vi "Grid_Move_to_point.vi"(6 "point":i64, 9 "FileRefs in":T1, 10 "Settings":T2={"Drift Correction Settings"={"Drift Correction every"=80, "Drift correction Pixels"=256, "Channel index (0-23)"=0, "MaxImagesBack"=2, "Threshold"=2, "Increment"=8, "max applied Drift Correction"=20, "Correct Drift"=TRUE, "Correlate"=0, "Correct z drift"=FALSE, "zdrift \nDuration (s)"=0.0}, "Spectroscopy Setting"={"Imaging Current"=1e-11, "ref Current"=7e-11, "tip Speed (m/s)"=2e-09, "Imaging Bias"=0.02, "ref Bias"=-0.1, "preSTS delay [ms]"=500, "STS z offset"=2e-10, "during Spec Bias (V)"=-0.1, "trigger1 < Hz"=0.0, "trigger 2 >Hz"=0.0, "autoStop"=FALSE, "Spectroscopy"=0, "PLL ON/OFF"=TRUE, "readjust setpoint every "=1, "z Reference"=FALSE, "Lock In"=TRUE}, "Misc"={"File name"="symmetric_node_zOff=200p", "Email when finished"="cornelius.krull@monash.edu,Dhaneesh.Gopalakrishnan@monash.edu,marina.castelli@monash.edu"}, "Grid Settings"={"type"=1, "type order"=1, "X pixel"=0, "Y pixel"=0, "Grid_Parms"={"center X (m)"=0.0, "center Y (m)"=0.0, "width (m)"=0.0, "height (m)"=0.0, "angle (deg)"=0.0}}} {"Grid Settings"."type order" items=["Line", "Grid"]; "Grid Settings"."type" items=["Line", "Grid"]; "Spectroscopy Setting"."Spectroscopy" items=["Bias", "zSpec"]; "Spectroscopy Setting"."trigger 2 >Hz" format="%#_6p"; "Spectroscopy Setting"."trigger1 < Hz" format="%#_6p"; "Spectroscopy Setting"."during Spec Bias (V)" format="%#_5p"; "Spectroscopy Setting"."STS z offset" format="%#_6p"; "Spectroscopy Setting"."ref Bias" format="%#_6p"; "Spectroscopy Setting"."Imaging Bias" format="%#_6p"; "Spectroscopy Setting"."tip Speed (m/s)" format="%.2p"; "Spectroscopy Setting"."ref Current" format="%#_6p"; "Spectroscopy Setting"."Imaging Current" format="%#_6p"; "Drift Correction Settings"."Correlate" items=["first Frame", "successive Frames"]; "Drift Correction Settings"."max applied Drift Correction" min=1 max=100 step=1 format="%.0p"; "Drift Correction Settings"."Threshold" min=1 step=1; "Drift Correction Settings"."Channel index (0-23)" items=["Current"=0, "Z (m)"=14]}, 11 "Application ref in":refnum<vi>) -> (1 "FileRefs out":T1, 2 "Settings out":T2={"Drift Correction Settings"={"Drift Correction every"=80, "Drift correction Pixels"=256, "Channel index (0-23)"=0, "MaxImagesBack"=2, "Threshold"=2, "Increment"=8, "max applied Drift Correction"=20, "Correct Drift"=TRUE, "Correlate"=0, "Correct z drift"=FALSE, "zdrift \nDuration (s)"=0.0}, "Spectroscopy Setting"={"Imaging Current"=1e-11, "ref Current"=7e-11, "tip Speed (m/s)"=2e-09, "Imaging Bias"=0.02, "ref Bias"=-0.1, "preSTS delay [ms]"=500, "STS z offset"=2e-10, "during Spec Bias (V)"=-0.1, "trigger1 < Hz"=0.0, "trigger 2 >Hz"=0.0, "autoStop"=FALSE, "Spectroscopy"=0, "PLL ON/OFF"=TRUE, "readjust setpoint every "=1, "z Reference"=FALSE, "Lock In"=TRUE}, "Misc"={"File name"="symmetric_node_zOff=200p", "Email when finished"="cornelius.krull@monash.edu,Dhaneesh.Gopalakrishnan@monash.edu,marina.castelli@monash.edu"}, "Grid Settings"={"type"=1, "type order"=1, "X pixel"=0, "Y pixel"=0, "Grid_Parms"={"center X (m)"=0.0, "center Y (m)"=0.0, "width (m)"=0.0, "height (m)"=0.0, "angle (deg)"=0.0}}} {"Grid Settings"."type order" items=["Line", "Grid"]; "Grid Settings"."type" items=["Line", "Grid"]; "Spectroscopy Setting"."Spectroscopy" items=["Bias", "zSpec"]; "Spectroscopy Setting"."trigger 2 >Hz" format="%#_6p"; "Spectroscopy Setting"."trigger1 < Hz" format="%#_6p"; "Spectroscopy Setting"."during Spec Bias (V)" format="%#_5p"; "Spectroscopy Setting"."STS z offset" format="%#_6p"; "Spectroscopy Setting"."ref Bias" format="%#_6p"; "Spectroscopy Setting"."Imaging Bias" format="%#_6p"; "Spectroscopy Setting"."tip Speed (m/s)" format="%.2p"; "Spectroscopy Setting"."ref Current" format="%#_6p"; "Spectroscopy Setting"."Imaging Current" format="%#_6p"; "Drift Correction Settings"."Correlate" items=["first Frame", "successive Frames"]; "Drift Correction Settings"."max applied Drift Correction" min=1 max=100 step=1 format="%.0p"; "Drift Correction Settings"."Threshold" min=1 step=1; "Drift Correction Settings"."Channel index (0-23)" items=["Current"=0, "Z (m)"=14]}, 3 "Application ref out":refnum<vi>)   [LabVIEW 2021]
uses:
  <userlib>/Nanonis Prog Interface V5/Scan/Grid/CloudPatternGet.vi
  <userlib>/Nanonis Prog Interface V5/Nanonis Prog Interface.lvlib
panel:
  out "error out":errorcluster
  in  "error in":errorcluster
  # "z Spectroscopy"
  # "GRID points"
  # "Increase this if no Drift was detected for \na certain number of images"
  # "% of image size"
  # "z Spectroscopy"
  # "GRID points"
  # "Increase this if no Drift was detected for \na certain number of images"
  # "% of image size"
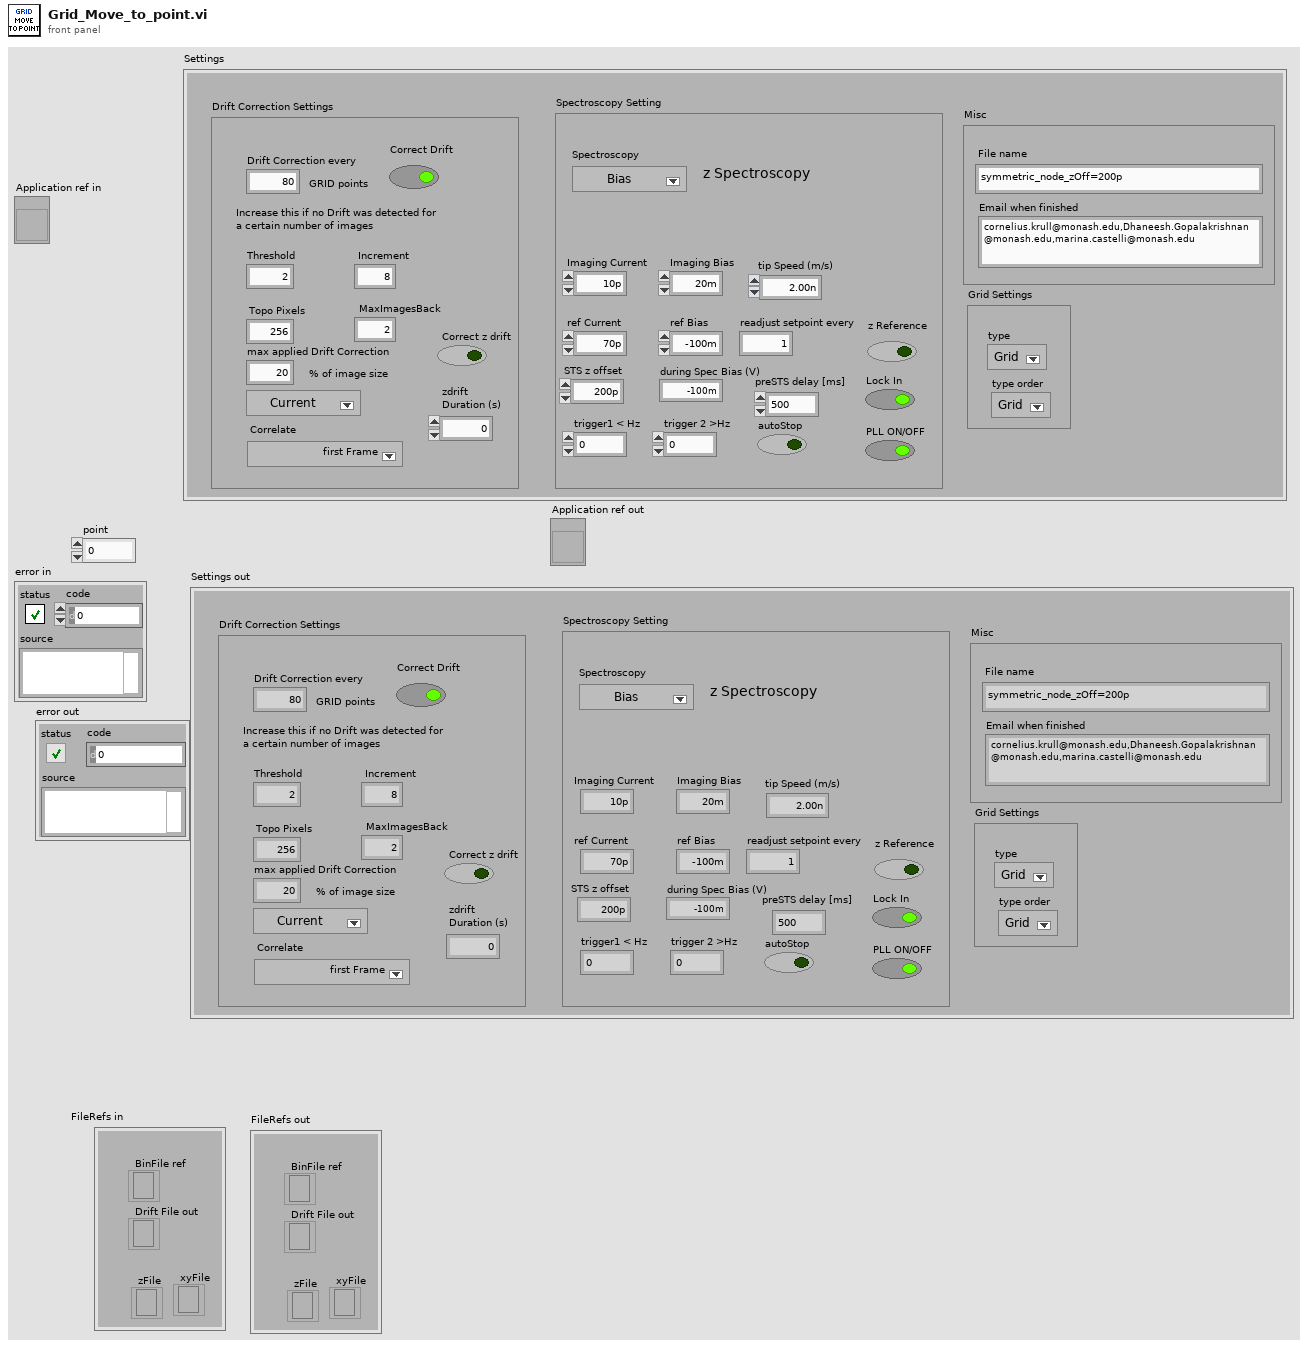
[diagram p1: front panel]
types:
  T1 = cluster{"Drift File out":refnum<file>, "zFile":refnum<file>, "BinFile ref":refnum<file>, "xyFile":refnum<file>}
  T2 = cluster{"Drift Correction Settings":cluster{"Drift Correction every":i32, "Drift correction Pixels":i32, "Channel index (0-23)":u8, "MaxImagesBack":i32, "Threshold":i32, "Increment":i32, "max applied Drift Correction":i32, "Correct Drift":bool, "Correlate":u16, "Correct z drift":bool, "zdrift \nDuration (s)":dbl}, "Spectroscopy Setting":cluster{"Imaging Current":dbl, "ref Current":dbl, "tip Speed (m/s)":sgl, "Imaging Bias":dbl, "ref Bias":dbl, "preSTS delay [ms]":u32, "STS z offset":dbl, "during Spec Bias (V)":sgl, "trigger1 < Hz":sgl, "trigger 2 >Hz":sgl, "autoStop":bool, "Spectroscopy":u16, "PLL ON/OFF":bool, "readjust setpoint every ":i32, "z Reference":bool, "Lock In":bool}, "Misc":cluster{"File name":string, "Email when finished":string}, "Grid Settings":cluster{"type":u16, "type order":u16, "X pixel":i32, "Y pixel":i32, "Grid_Parms":cluster{"center X (m)":sgl, "center Y (m)":sgl, "width (m)":sgl, "height (m)":sgl, "angle (deg)":sgl}}}
  T3 = cluster{"type":u16, "type order":u16, "X pixel":i32, "Y pixel":i32, "Grid_Parms":cluster{"center X (m)":sgl, "center Y (m)":sgl, "width (m)":sgl, "height (m)":sgl, "angle (deg)":sgl}}
  T4 = cluster{"type":u16, "type order":u16, "X pixel":dbl, "Y pixel":dbl, "Grid_Parms":cluster{"center X (m)":sgl, "center Y (m)":sgl, "width (m)":sgl, "height (m)":sgl, "angle (deg)":sgl}}
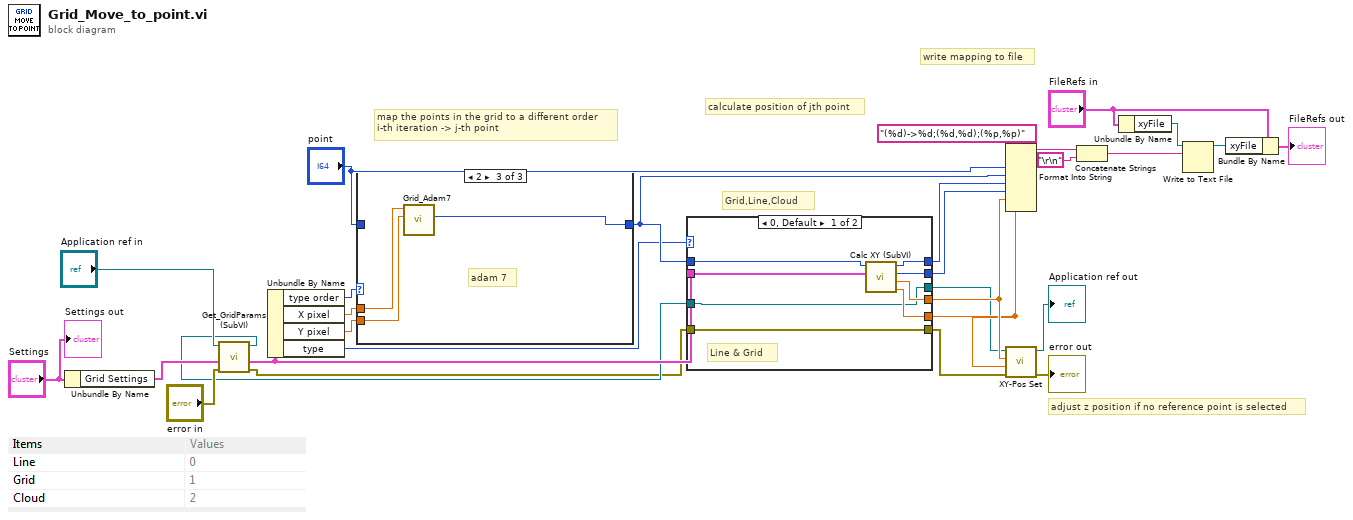
[diagram p0: block diagram]
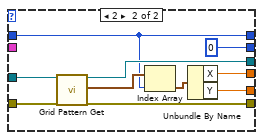
[diagram p2: hidden frame]
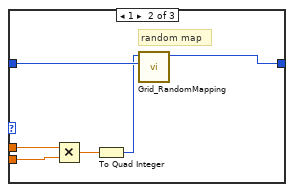
[diagram p4: hidden frame]
diagram:
  # "Grid,Line,Cloud"
  # "adjust z position if no reference point is selected"
  # "calculate position of jth point"
  # "write mapping to file"
  # "map the points in the grid to a different order\ni-th iteration -> j-th point"
  n1 = Unbundle By Name("Settings") -> ("Grid Settings"=w29:T3)
  n2 = call "Get_GridParams (SubVI).vi"("error in (no error)"="error in", "Grid Settings"=w29, "Application in"="Application ref in") -> ("error out"=w2:errorcluster, "Grid Settings"=w12:T4, "Application out"=w4:refnum<vi>)  [unwired: 5 in, 1 out]
  n3 = Unbundle By Name(w12) -> ("type order"=w13:u16, "X pixel"=w10:dbl, "Y pixel"=w11:dbl, "type"=w5:u16)
  n4 = case shown="2" w13 {
    tunnel: "point" -> [w30 w36 _]
    tunnel: [w30 w35 w39] -> w21
    tunnel: w11 -> [_ w33 w37]
    tunnel: w10 -> [_ w32 w38]
    frame 0, Default {
      # "standard bottom left to top right"
    }
    frame 1 {
      # "random map"
      n5 = Multiply(x=w32, y=w33) -> (x*y=w34:dbl)
      n6 = To Quad Integer(1:w34) -> (0:w31:i64)
      n7 = call "Grid_RandomMapping.vi"("Point"=w36, "NumPoints"=w31) -> ("element"=w35:i64)  [unwired: 9 in]
    }
    frame 2 {
      # "adam 7"
      n8 = call "Grid_Adam7.vi"("py 2"=w37, "px 2"=w38) -> ("index of element"=w39:i32)  [unwired: 8 in, 1 out]
    }
  }
  n9 = case shown="0, Default" w5 {
    tunnel: w21 -> [w47 w49]
    tunnel: [w46 w49] -> w20
    tunnel: [w45 i64 0 ("y_i")] -> w19
    tunnel: w12 -> [w44 _]
    tunnel: [w43 w51] -> w7
    tunnel: [w42 w50] -> w6
    tunnel: w4 -> [w41 w57]
    tunnel: [w41 w56] -> w3
    tunnel: w2 -> [w40 w55]
    tunnel: [w40 w54] -> w1
    frame 0, Default {
      # "Line & Grid"
      n10 = call "Calc XY (SubVI).vi"("Grid Settings"=w44, "element"=w47) -> ("y2"=w42:dbl, "x2"=w43:dbl, "y_i"=w45:i64, "x_i"=w46:i64)  [unwired: 6 in]
    }
    frame 2 {
      n11 = call-poly <userlib>:"Grid Pattern Get.vi"("Application ref in"=w57, "error in (no error)"=w55) -> ("Application ref out"=w56:refnum<vi>, "Cloud data"=w53:cluster{"X":sgl, "Y":sgl}[], "error out"=w54:errorcluster)  [unwired: 15 in]
      n12 = Index Array(array=w53, index=w49) -> (element=w52:cluster{"X":sgl, "Y":sgl})
      n13 = Unbundle By Name(w52) -> ("X"=w51:sgl, "Y"=w50:sgl)
    }
  }
  n14 = Format Into String(format string="(%d)->%d;(%d,%d);(%p,%p)", "point", w21, w20, w19, w7, w6) -> (resulting string=w18:string)  [unwired: 2 in, 1 out]
  n15 = call <userlib>:"XY-Pos Set.vi"("error in (no error)"=w1, "Y (m)"=w6, "X (m)"=w7, "Application ref in"=w3) -> ("error out"=→"error out":errorcluster, "Application ref out"=→"Application ref out":refnum<vi>)  [unwired: 4 in]
  n16 = Concatenate Strings(w18, "\r\n") -> (w9:string)
  n17 = Unbundle By Name("FileRefs in") -> ("xyFile"=w26:refnum<file>)
  n18 = Write to Text File(file (use dialog)=w26, text=w9) -> (refnum out=w24:refnum<file>)  [unwired: 2 in, 2 out]
  n19 = Bundle By Name(cluster="FileRefs in", "xyFile"=w24) -> (→"FileRefs out":T1)
  "Settings out" <- "Settings"
